vi "Command Finished.vi"(8 "error in (no error)":errorcluster, 11 "No Command in":refnum<class "No Command.lvclass">) -> (0 "error out":errorcluster, 3 "No Command out":refnum<class "No Command.lvclass">)   [LabVIEW 2013, in "Robot Actors.lvlib" / "Command Processor.lvlib" / "No Command.lvclass"]
uses:
  No Command.lvclass
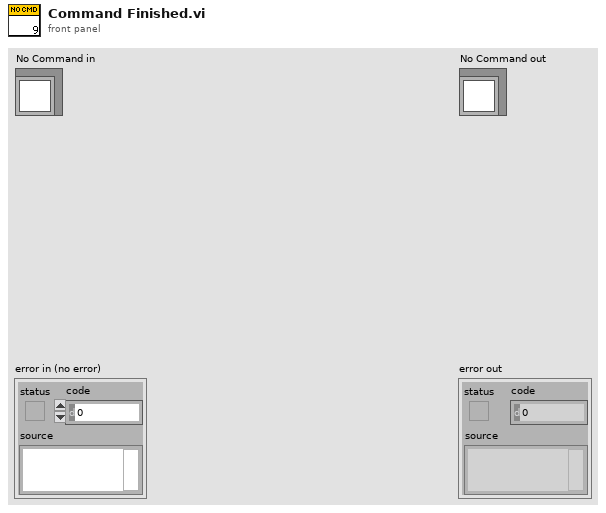
[diagram p1: front panel]
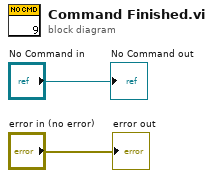
[diagram p0: block diagram]
diagram:
  "error out" <- "error in (no error)"
  "No Command out" <- "No Command in"
